vi "Holding Register Set Mapping.vi"(8 "error in (no error)":errorcluster, 10 "Mapping":T2, 11 "Item Ref in":T1 format="%.0x") -> (0 "error out":errorcluster, 3 "Item Ref out":T1 format="%.0x")   [LabVIEW 2015, in "Modbus Master System Explorer.lvlib"]
uses:
  Modbus Master System Explorer.lvlib
  <vilib>/NI Veristand/Custom Device API/Custom Device Item Ref.ctl
  Shared/Controls/Data Model/Mapping.ctl
  Shared/Controls/Data Model/DataType.ctl
  <vilib>/NI VeriStand/Custom Device API/Custom Device API.lvlib
  Shared/Modbus Master Shared.lvlib
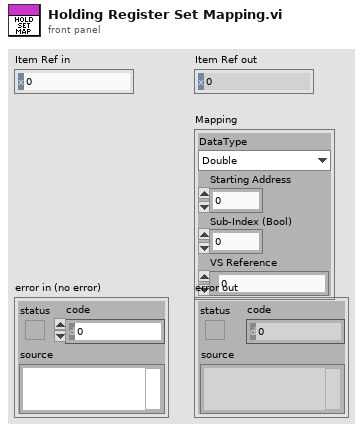
[diagram p1: front panel]
types:
  T1 = typedef "Custom Device API.lvlib/Custom Device Item Ref.ctl" = u64
  T2 = typedef "Modbus Master Shared.lvlib/Mapping.ctl" = cluster{"DataType":T3, "Starting Address":u16, "Sub-Index (Bool)":u16, "VS Reference":T1}
  T3 = typedef "Modbus Master Shared.lvlib/DataType.ctl" = enum16{"Double", "Single", "I64", "I32", "I16", "I8", "U64", "U32", "U16", "U8", "Boolean"}
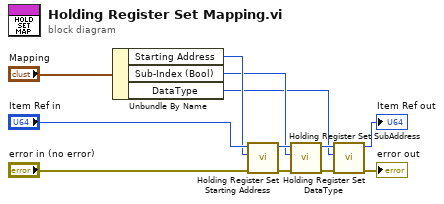
[diagram p0: block diagram]
diagram:
  n1 = Unbundle By Name("Mapping") -> ("Starting Address"=w8:u16, "Sub-Index (Bool)"=w7:u16, "DataType"=w6:T3)
  n2 = call "Holding Register Set Starting Address.vi"("error in (no error)"="error in (no error)", "Value"=w8, "Item Ref in"="Item Ref in") -> ("error out"=w4:errorcluster, "Item Ref out"=w11:T1)  [unwired: 7 in]
  n3 = call "Holding Register Set SubAddress.vi"("error in (no error)"=w4, "Value"=w7, "Item Ref in"=w11) -> ("error out"=w5:errorcluster, "Item Ref out"=w12:T1)  [unwired: 7 in]
  n4 = call "Holding Register Set DataType.vi"("error in (no error)"=w5, "DataType"=w6, "Item Ref in"=w12) -> ("error out"=→"error out":errorcluster, "Item Ref out"=→"Item Ref out":T1)  [unwired: 7 in]
